vi "Control References.vi"() -> ()   [LabVIEW 2019]
doc: "Demonstrates the use of Control References to manipulate front panel objects.\n\n1) Uses implicitly linked Property Nodes, which you can create by right-clicking a control or indicator and selecting <B>Create>>Property Node</B> from the shortcut menu. This approach does not use control references.\n\n2) Uses control references, which you can create by right-clicking a control or indicator and selecting <B>Create»Reference</B> from the shortcut menu. You can wire the control reference to the reference input of a Property Node or Invoke Node.\n\n3) Passes a control reference to a subVI."
panel:
  in  "Change Visibility":bool
  in  "Selected Control":enum32{"Boolean", "String"}(radio)
  in  "Stop":bool
  in  "Y Scale.Range:Maximum":dbl=100.0 format="%#.6g"
  in  "Y Scale.Range:Minimum":dbl format="%#.6g"
  out "Waveform Chart":dbl(graph)
  in  "String":string
  in  "Boolean":bool
  in  "Disabled Status":u16(ring) items=["Enabled", "Disabled", "Disabled and Grayed Out"]
  in  "Numeric":dbl format="%#.6g"
  # "Overview: Demonstrates the use of the Control References to programmatically manipulate front panel objects through VI Server.\nInstructions:\n1. Run the VI.\n2. Change the Disabled Status value to enable/disable the Numeric control.\n3. Click the Change Visibility button to show/hide the Selected Control.\n4. Change the Minimum and Maximum values of the Y Scale of the Waveform Chart.\n5. Click Stop to stop the VI. See the diagram for more information on using control references to manipulate front panel objects."
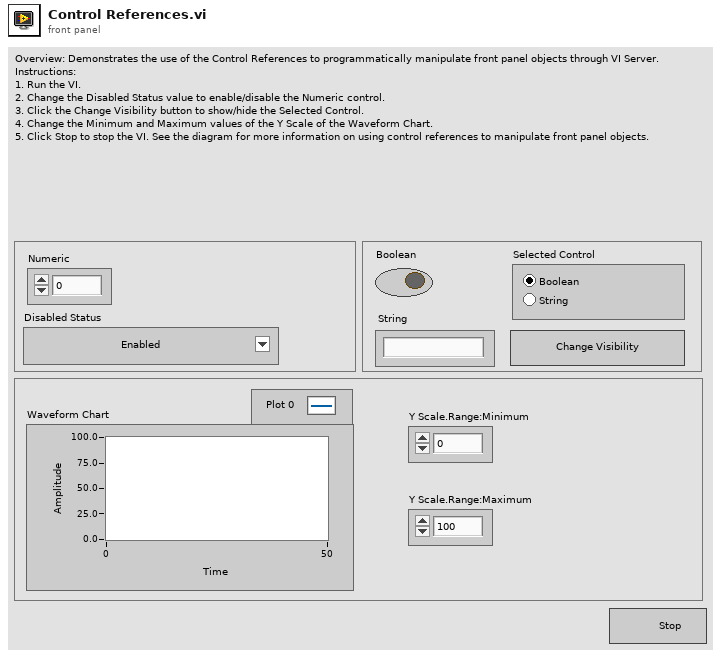
[diagram p1: front panel]
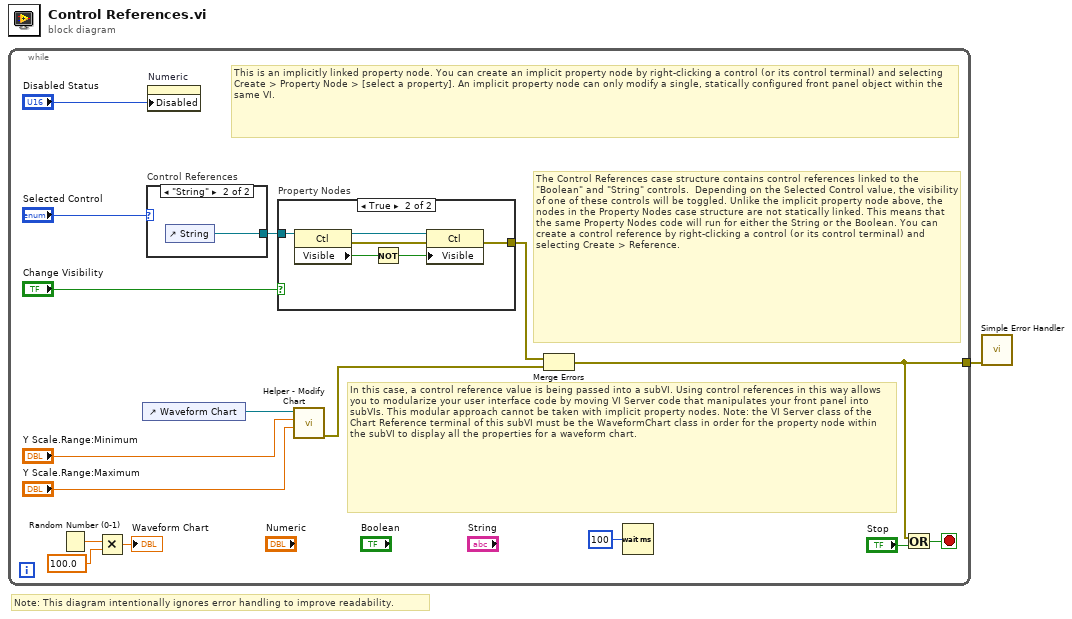
[diagram p0: block diagram]
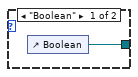
[diagram p3: hidden frame]
diagram:
  # "Note: This diagram intentionally ignores error handling to improve readability."
  n1 = while {
    tunnel: [w2] -> w1
    stop <- w3 stop-if-true
    # "In this case, a control reference value is being passed into a subVI. Using control references in this way allows you to modularize your user interface code by moving VI Server code that manipulates your front panel into subVIs. This modular approach cannot be taken with implicit property nodes. Note: the VI Server class of the Chart Reference terminal of this subVI must be the WaveformChart class in order for the property node within the subVI to display all the properties for a waveform chart."
    # "The Control References case structure contains control references linked to the \"Boolean\" and \"String\" controls.  Depending on the Selected Control value, the visibility of one of these controls will be toggled. Unlike the implicit property node above, the nodes in the Property Nodes case structure are not statically linked. This means that the same Property Nodes code will run for either the String or the Boolean. You can create a control reference by right-clicking a control (or its control terminal) and selecting Create > Reference."
    # "This is an implicitly linked property node. You can create an implicit property node by right-clicking a control (or its control terminal) and selecting Create > Property Node > [select a property]. An implicit property node can only modify a single, statically configured front panel object within the same VI."
    n2 = Random Number (0-1)() -> (number: 0 to 1=w13:dbl)
    n3 = Multiply(x=w13, y=100.0) -> (x*y=→"Waveform Chart":dbl)
    n4 = control-ref of="Waveform Chart"() -> (w16:refnum<vi>)
    n5 = case "Control References" shown="\"String\"" "Selected Control" {
      tunnel: [w24 w25] -> w7
      frame "Boolean" {
        n6 = control-ref of="Boolean"() -> (w24:refnum<vi>)
      }
      frame "String" {
        n7 = control-ref of="String"() -> (w25:refnum<vi>)
      }
    }
    n8 = property on="Numeric" class="DigNum (strict)"("Disabled"="Disabled Status") -> ()  [unwired: 2 in, 2 out]
    n9 = case "Property Nodes" shown="True" "Change Visibility" {
      tunnel: w7 -> [_ w23]
      tunnel: [_ w18] -> w5
      frame False {
      }
      frame True {
        n10 = property class="Ctl"(reference=w23) -> (reference out=w22:refnum<vi>, error out=w21:errorcluster, "Visible"=w20:bool)  [unwired: 1 in]
        n11 = Not(x=w20) -> (.not. x?=w19:bool)
        n12 = property class="Ctl"(reference=w22, error in=w21, "Visible"=w19) -> (error out=w18:errorcluster)  [unwired: 1 out]
      }
    }
    n13 = call "Helper - Modify Chart.vi"("Y Scale.Range:Maximum"="Y Scale.Range:Maximum", "Y Scale.Range:Minimum"="Y Scale.Range:Minimum", "Chart Reference"=w16) -> ("error out"=w4:errorcluster)  [unwired: 8 in]
    n14 = Merge Errors(w5, w4) -> (w2:errorcluster)
    n15 = Wait (ms)(milliseconds to wait=u32 100 ("millisecond timer value")) -> ()  [unwired: 1 out]
    n16 = Or(x=w2, y="Stop") -> (x .or. y?=w3:bool)
  }
  n17 = call <vilib>:"Simple Error Handler.vi"("error in (no error)"=w1) -> ()  [unwired: 4 in, 5 out]
